vi "Register gRPC Methods.vi"(8 "error in (no error)":errorcluster, 11 "Template Server in":refnum<class "HVC7.lvclass">) -> (0 "error out":errorcluster, 3 "Template Server out":refnum<class "HVC7.lvclass">)   [LabVIEW 2019, in "HVC7.lvlib" / "HVC7.lvclass"]
uses:
  HVC7.lvclass
  typeDefs/Server Internal UEs.ctl
  typeDefs/Server Internal Message.ctl
  typeDefs/Server gRPC UEs.ctl
  gRPC lvSupport/Server API/typeDefs/gRPCId Cluster.ctl
  gRPC lvSupport/Server API/typeDefs/grpcId.ctl
  HVC7.lvclass/HVC7.ctl
  gRPC lvSupport/gprc-lvsupport.lvlib
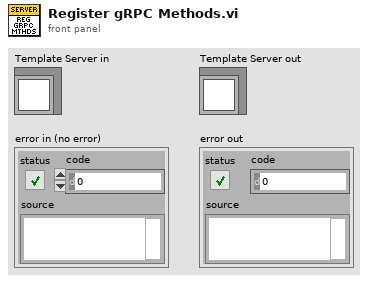
[diagram p1: front panel]
types:
  T1 = typedef "HVC7.lvlib/HVC7.lvclass/Server gRPC UEs.ctl" = cluster{"Invoke gRPC UE":refnum<user-event>, "Query gRPC UE":refnum<user-event>, "Register gRPC UE":refnum<user-event>, "OpenDIOSession gRPC UE":refnum<user-event>, "ReadDI gRPC UE":refnum<user-event>, "WriteDO gRPC UE":refnum<user-event>, "CloseDIOSession gRPC UE":refnum<user-event>}
  T2 = typedef "HVC7.lvlib/HVC7.lvclass/Server Internal UEs.ctl" = cluster{"Invoke Internal UE":refnum<user-event>, "Query Internal UE":refnum<user-event>, "Register Internal UE":refnum<user-event>, "OpenDIOSession Internal UE":refnum<user-event>, "ReadDI Internal UE":refnum<user-event>, "WriteDO Internal UE":refnum<user-event>, "CloseDIOSession Internal UE":refnum<user-event>}
  T3 = typedef "HVC7.lvlib/gprc-lvsupport.lvlib/grpcId.ctl" = u64
  T4 = typedef "HVC7.lvlib/HVC7.lvclass/Server Internal Message UE.ctl" = refnum<user-event>
  T5 = typedef "HVC7.lvlib/gprc-lvsupport.lvlib/gRPCId Cluster UE.ctl" = refnum<user-event>
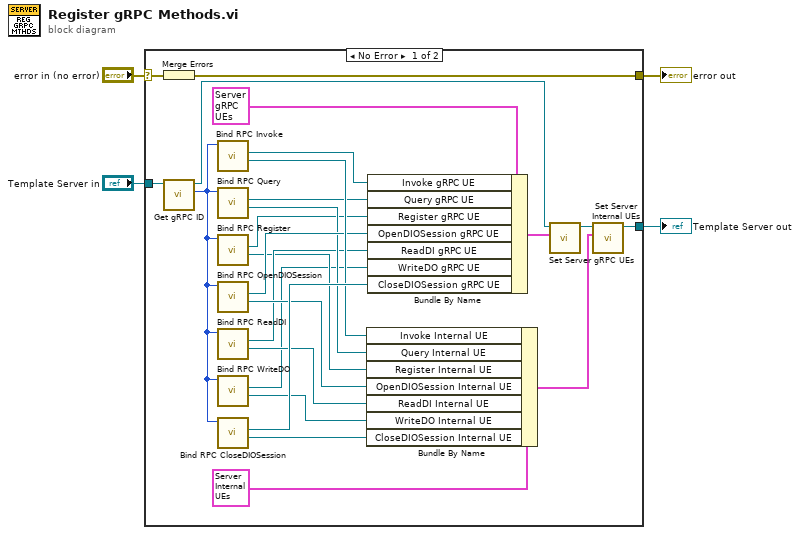
[diagram p0: block diagram]
diagram:
  n1 = case shown="No Error" "error in (no error)" {
    selector: "error in (no error)" -> [w20 w30]
    tunnel: "Template Server in" -> [w28 w31]
    tunnel: [w27 w30] -> w3
    tunnel: [w26 w31] -> w2
    frame No Error {
      n2 = Merge Errors(w20) -> (w27:errorcluster)
      n3 = call "Get gRPC ID.vi"("OOP Server in"=w28) -> ("gRPC ID"=w19:T3, "OOP Server out"=w29:refnum<class "HVC7.lvclass">)  [unwired: 9 in]
      n4 = call "Bind RPC Invoke.vi"("gRPCid server in"=w19) -> ("Invoke Internal UE"=w16:T4, "Invoke gRPC UE"=w15:T5)  [unwired: 7 in, 2 out]
      n5 = call "Bind RPC Query.vi"("gRPCid server in"=w19) -> ("Query Internal UE"=w12:T4, "Query gRPC UE"=w11:T5)  [unwired: 7 in, 2 out]
      n6 = call "Bind RPC Register.vi"("gRPCid server in"=w19) -> ("Register Internal UE"=w8:T4, "Register gRPC UE"=w7:T5)  [unwired: 7 in, 2 out]
      n7 = call "Bind RPC OpenDIOSession.vi"("gRPCid server in"=w19) -> ("OpenDIOSession Internal UE"=w14:T4, "OpenDIOSession gRPC UE"=w13:T5)  [unwired: 7 in, 2 out]
      n8 = call "Bind RPC ReadDI.vi"("gRPCid server in"=w19) -> ("ReadDI Internal UE"=w10:T4, "ReadDI gRPC UE"=w9:T5)  [unwired: 7 in, 2 out]
      n9 = call "Bind RPC WriteDO.vi"("gRPCid server in"=w19) -> ("WriteDO Internal UE"=w6:T4, "WriteDO gRPC UE"=w5:T5)  [unwired: 7 in, 2 out]
      n10 = call "Bind RPC CloseDIOSession.vi"("gRPCid server in"=w19) -> ("CloseDIOSession Internal UE"=w18:T4, "CloseDIOSession gRPC UE"=w17:T5)  [unwired: 7 in, 2 out]
      n11 = Bundle By Name ("Bundle Internal UEs")(cluster=T2 {"Invoke Internal UE"=refnum, "Query Internal UE"=refnum, "Register Internal UE"=refnum, "OpenDIOSession Internal UE"=refnum, "ReadDI Internal UE"=refnum, "WriteDO Internal UE"=refnum, "CloseDIOSession Internal UE"=refnum} ("Server Internal UEs"), "Invoke Internal UE"=w16, "Query Internal UE"=w12, "Register Internal UE"=w8, "OpenDIOSession Internal UE"=w14, "ReadDI Internal UE"=w10, "WriteDO Internal UE"=w6, "CloseDIOSession Internal UE"=w18) -> (w25:T2)
      n12 = Bundle By Name ("Bundle gRPC UEs")(cluster=T1 {"Invoke gRPC UE"=refnum, "Query gRPC UE"=refnum, "Register gRPC UE"=refnum, "OpenDIOSession gRPC UE"=refnum, "ReadDI gRPC UE"=refnum, "WriteDO gRPC UE"=refnum, "CloseDIOSession gRPC UE"=refnum} ("gRPC Server Method Events"), "Invoke gRPC UE"=w15, "Query gRPC UE"=w11, "Register gRPC UE"=w7, "OpenDIOSession gRPC UE"=w13, "ReadDI gRPC UE"=w9, "WriteDO gRPC UE"=w5, "CloseDIOSession gRPC UE"=w17) -> (w22:T1)
      n13 = call "Set Server gRPC UEs.vi"("Server gRPC UEs"=w22, "OOP Server in"=w29) -> ("OOP Server out"=w23:refnum<class "HVC7.lvclass">)  [unwired: 9 in]
      n14 = call "Set Server Internal UEs.vi"("Server Internal UEs"=w25, "OOP Server in"=w23) -> ("OOP Server out"=w26:refnum<class "HVC7.lvclass">)  [unwired: 9 in]
    }
    frame Error {
    }
  }
  "error out" <- w3
  "Template Server out" <- w2
